vi "Stop Receiving.vi"(8 "error in (no error)":errorcluster, 11 "Vision in":refnum<class "Vision.lvclass">) -> (0 "error out":errorcluster, 3 "Vision out":refnum<class "Vision.lvclass">)   [LabVIEW 2022 SP3, in "Vision.lvlib" / "Vision.lvclass"]
uses:
  Vision.lvclass
  Vision.lvclass/Vision.ctl
  UDP Data Receiver/UDP Data Receiver Messages/Stop Receiving Msg/Stop Receiving Msg.lvclass
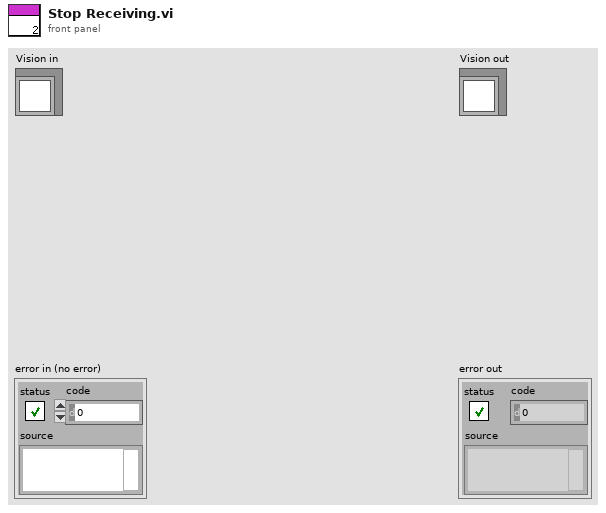
[diagram p1: front panel]
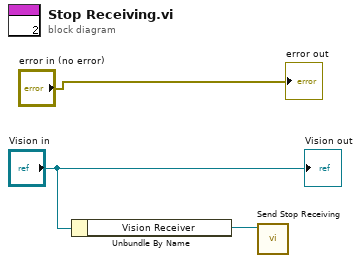
[diagram p0: block diagram]
diagram:
  n1 = Unbundle By Name("Vision in") -> ("Vision Receiver"=w1:refnum<class "Message Enqueuer.lvclass">)
  n2 = call "Send Stop Receiving.vi"("Message Enqueuer"=w1) -> ()  [unwired: 9 in, 2 out]
  "error out" <- "error in (no error)"
  "Vision out" <- "Vision in"
